vi "FRCts20_Backend_Error_To_Status - Multiple.vi"(10 "error in (no error)":errorcluster, 11 "rows affected?":bool) -> (2 "error out":errorcluster, 3 "String":string)   [LabVIEW 2014, in "FRCts20_Backend_Engine.lvlib"]
doc: "This Vi takes the number of rows affected by an sql command and the error returned, and converts that to a status message. That is, if there was no error and many rows were affected, we get a \"success\", while 0 rows affected or an error message is a failure."
uses:
  FRCts20_Backend_Engine.lvlib
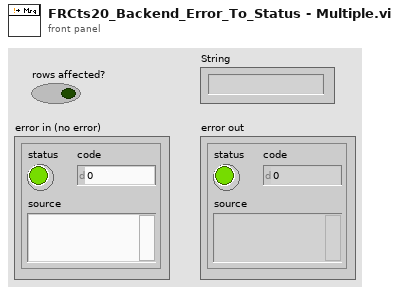
[diagram p1: front panel]
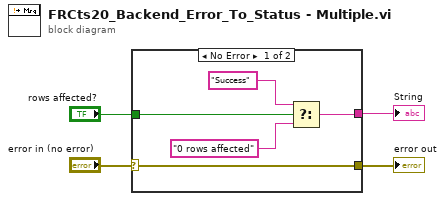
[diagram p0: block diagram]
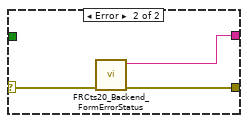
[diagram p2: hidden frame]
diagram:
  n1 = case shown="No Error" "error in (no error)" {
    selector: "error in (no error)" -> [w9 w11]
    tunnel: [w9 w12] -> w2
    tunnel: [w8 w10] -> w4
    tunnel: "rows affected?" -> [w5 _]
    frame No Error {
      n2 = Select(t="Success", s=w5, f="0 rows affected") -> (s? t:f=w8:string)
    }
    frame Error {
      n3 = call "FRCts20_Backend_FormErrorStatus.vi"("error in (no error)"=w11) -> ("error out"=w12:errorcluster, "String"=w10:string)  [unwired: 9 in]
    }
  }
  "String" <- w4
  "error out" <- w2
